vi "getTaskReference.vi"(8 "error in (no error)":errorcluster, 11 "ExampleTask_StopNotifier in":refnum<class "Task_BoolUserEventStopMech.lvclass">) -> (0 "error out":errorcluster, 2 "taskRef":refnum<vi>, 3 "ExampleTask_StopNotifier out":refnum<class "Task_BoolUserEventStopMech.lvclass">)   [LabVIEW 2023, in "Task_BoolUserEventStopMech.lvclass"]
doc: "Returns the VI reference related to the task to handle.\n_____________________________________\nTLC Daemon 1.0.0.2\nCopyright (c) 2026 Andrea Cadei"
uses:
  Task_BoolUserEventStopMech.lvclass
  myTask.vi
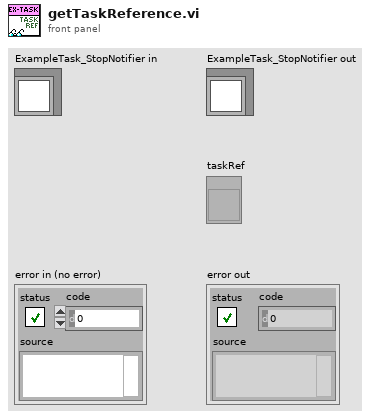
[diagram p1: front panel]
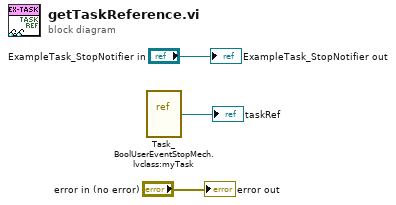
[diagram p0: block diagram]
diagram:
  n1 = vi-ref "Task_BoolUserEventStopMech.lvclass:myTask.vi"() -> (→"taskRef":refnum<vi>)
  "error out" <- "error in (no error)"
  "ExampleTask_StopNotifier out" <- "ExampleTask_StopNotifier in"
